vi "TCL Get Current Fragments - 1eventNfrag.vi"(3 "error in (no error)":errorcluster, 4 "fragments":string[](array[string]), 5 "event number":i32) -> (0 "error out":errorcluster, 1 "values":string[][](array[string]), 2 "fragments out":string[](array[string]))   [LabVIEW 2010]
uses:
  TCL Global.vi
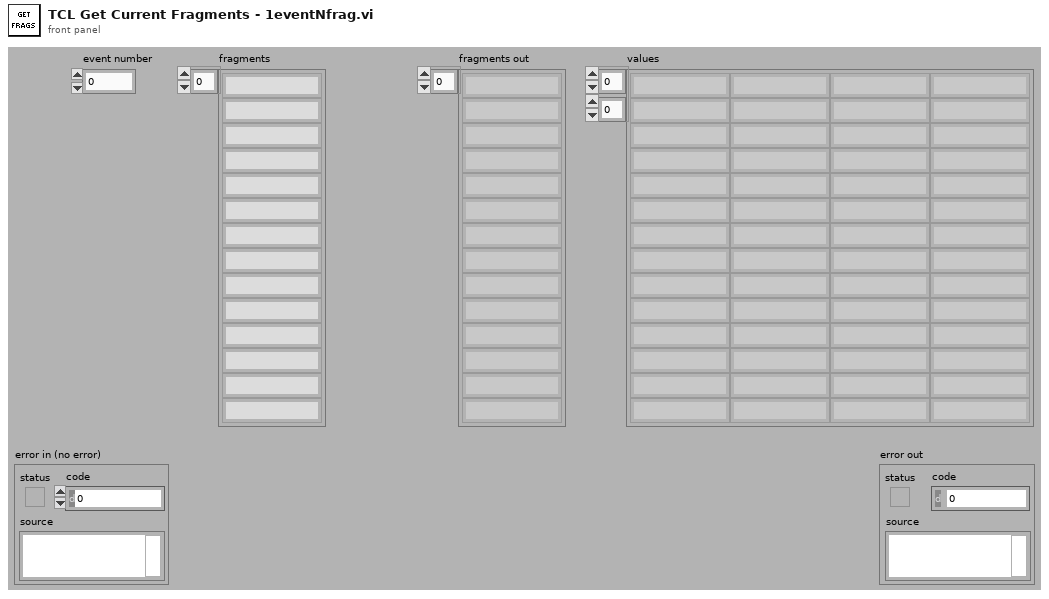
[diagram p1: front panel]
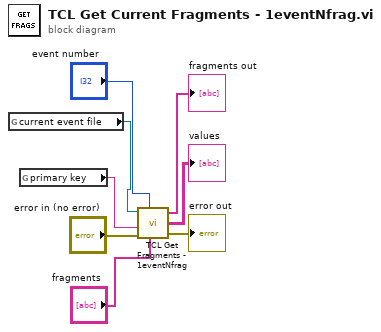
[diagram p0: block diagram]
diagram:
  n1 = global read "TCL Global.vi" "current event file"() -> (w1:path)
  n2 = global read "TCL Global.vi" "primary key"() -> (w2:string)
  n3 = call "TCL Get Fragments - 1eventNfrag.vi"("event file"=w1, "event number"="event number", "primary key"=w2, "fragments"="fragments", "error in (no error)"="error in (no error)") -> ("fragments out"=→"fragments out":string[], "values"=→"values":string[][], "error out"=→"error out":errorcluster)  [unwired: 1 in]
